vi "BME_DG_SetG08TriggerParameters.vi"(8 "error in (no error)":errorcluster, 10 "BME_SG08_Settings":T4={"V2 Trigger Settings"={"Trigger on MS Bus"=24, "Force Trigger (µs)"=0.0, "Gate Type"=TRUE, "Synchronize Gate"=FALSE}, "SG08_Settings"={"Gate Terminate"=TRUE, "Gate Level"=1.0, "Gate Delay (µs)"=0.0, "StepBackTime (µs)"=0.0, "Burst Counter"=0, "Trigger Divider"=1, "Trigger Multiplier"=4}} {"SG08_Settings"."StepBackTime (µs)" min=0.0 format="%.6f"; "SG08_Settings"."Gate Delay (µs)" format="%.3f"; "SG08_Settings"."Gate Level" min=-2.5 max=2.5 format="%.3g"; "V2 Trigger Settings"."Trigger on MS Bus" format="%04x" items=["Local Primary0x1"=1, "Local Secondary0x2"=2, "Local Force 0x4"=4, "Resynchronize 0x8"=8, "StepBackOnBus 0x10"=16, "StartOnBus 0x20"=32, "InhibitOnBus 0x40"=64, "LoadDataOnBus 0x80"=128]; "V2 Trigger Settings"."Force Trigger (µs)" min=0.0 format="%.6f"}, 11 "DG Number":i32) -> (0 "error out":errorcluster)   [LabVIEW 2009, in "POLARIS BME DG.lvlib"]
doc: "long Set_TriggerParameters(BOOL TriggerTerminate, double InternalClock, double TriggerLevel, unsigned long PresetValue, unsigned long GateDivider, BOOL PositiveGate, BOOL InternalTrigger, BOOL InternalArm, BOOL SoftwareTrigger, BOOL RisingEdge, BOOL StopOnPreset, BOOL ResetWhenDone, BOOL TriggerEnable, long DG_Number);"
uses:
  POLARIS BME DG.lvlib
  BME_DG_V2TriggerSettings.ctl
  MSBusSignals.ctl
  SG08_Settings.ctl
  BME DLL/DelayGenerator.dll
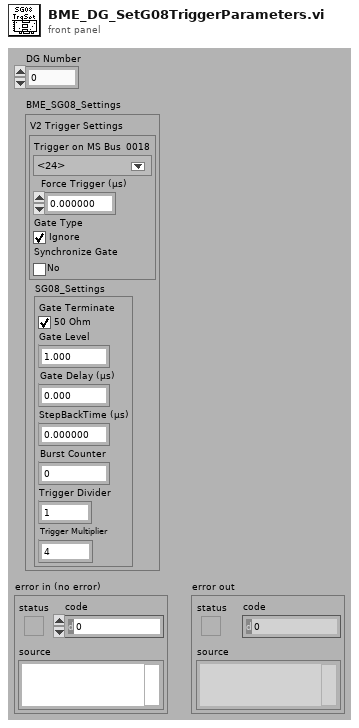
[diagram p1: front panel]
types:
  T1 = typedef "POLARIS BME DG.lvlib/BME_DG_V2TriggerSettings.ctl" = cluster{"Trigger on MS Bus":T2, "Force Trigger (µs)":dbl, "Gate Type":bool, "Synchronize Gate":bool}
  T2 = typedef "POLARIS BME DG.lvlib/MSBusSignals.ctl" = u32
  T3 = typedef "POLARIS BME DG.lvlib/SG08_Settings.ctl" = cluster{"Gate Terminate":bool, "Gate Level":dbl, "Gate Delay (µs)":dbl, "StepBackTime (µs)":dbl, "Burst Counter":u32, "Trigger Divider":u32, "Trigger Multiplier":u32}
  T4 = cluster{"V2 Trigger Settings":T1, "SG08_Settings":T3}
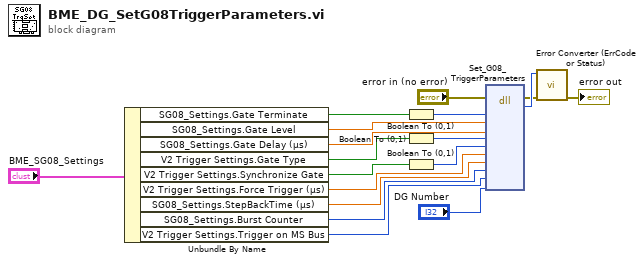
[diagram p0: block diagram]
diagram:
  n1 = Unbundle By Name("BME_SG08_Settings") -> ("SG08_Settings.Gate Terminate"=w7:bool, "SG08_Settings.Gate Level"=w10:dbl, "SG08_Settings.Gate Delay (µs)"=w9:dbl, "V2 Trigger Settings.Gate Type"=w5:bool, "V2 Trigger Settings.Synchronize Gate"=w4:bool, "V2 Trigger Settings.Force Trigger (µs)"=w8:dbl, "SG08_Settings.StepBackTime (µs)"=w11:dbl, "SG08_Settings.Burst Counter"=w12:u32, "V2 Trigger Settings.Trigger on MS Bus"=w13:T2)
  n2 = Boolean To (0,1)(Boolean=w7) -> (0, 1=w6:i16)
  n3 = Boolean To (0,1)(Boolean=w5) -> (0, 1=w2:i16)
  n4 = Boolean To (0,1)(Boolean=w4) -> (0, 1=w3:i16)
  n5 = dll-call lib="C:/CS Framework/LVSCC/LV2009/GPL/Projects/cs-framework/CSClass/CSPOLARIS/POLARIS BME DG/BME DLL/DelayGenerator.dll" fn="Set_G08_TriggerParameters"(error in="error in (no error)", "GateTerminate"=w6, "GateLevel"=w10, "GateDelay"=w9, "IgnoreGate"=w2, "SynchronizeGate"=w3, "ForceTrigger"=w8, "StepBackTime"=w11, "BurstCounter"=w12, "MS_Bus"=w13, "DG_Number"="DG Number") -> (error out=w16:errorcluster, "return type"=w18:i32)  [unwired: 12 in, 1 out]
  n6 = call "Error Converter (ErrCode or Status).vi"("error in (no error)"=w16, "error code"=w18) -> ("error out"=→"error out":errorcluster)  [unwired: 9 out]
